vi "Day.vi"() -> ()   [LabVIEW 2021]
uses:
  <vilib>/addons/_JKI Toolkits/Caraya/classes/Assert/Assert Equal Value_Variant.vi
  <vilib>/addons/_JKI Toolkits/Caraya/classes/Assert/Assert.lvclass
  <vilib>/addons/_JKI Toolkits/Caraya/classes/Test/Test.lvclass
panel:
  in  "Input?":enum16{"Examples", "File", "Web"}(ring)=enum."Web"
  in  "Part?":enum16{"Part 1", "Part 2"}(ring)
  out "Solution Part 2":i64
  out "Solution Part 1":i64
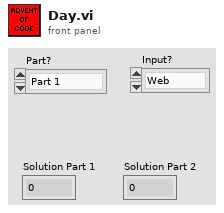
[diagram p1: front panel]
types:
  T1 = cluster{"Result Part1":dbl, "Result Part2":dbl, "Input":string}
  T2 = cluster{"Result Part1":dbl, "Result Part2":dbl, "Input":string}[]
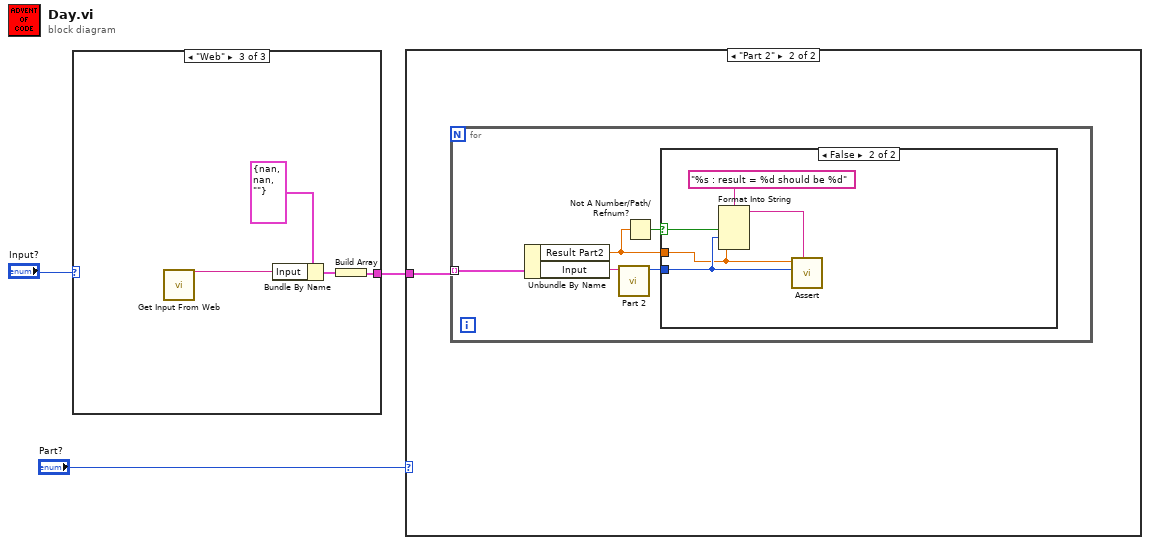
[diagram p0: block diagram]
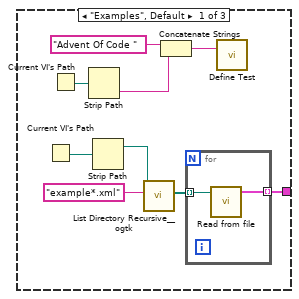
[diagram p2: hidden frame]
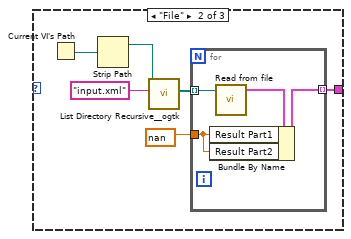
[diagram p3: hidden frame]
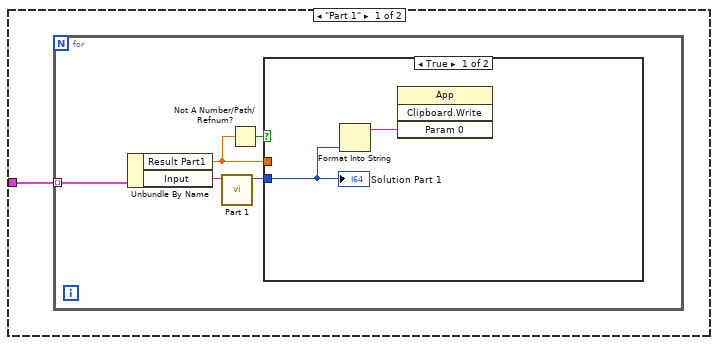
[diagram p4: hidden frame]
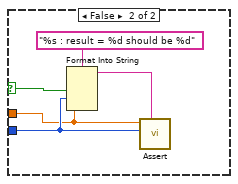
[diagram p5: hidden frame]
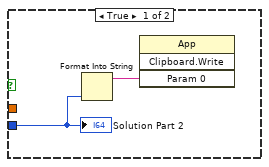
[diagram p6: hidden frame]
diagram:
  n1 = case shown="\"Web\"" "Input?" {
    tunnel: [w8 w16 w26] -> w1
    frame "Examples", Default {
      n2 = Current VI's Path() -> (path=w12:path)
      n3 = Current VI's Path() -> (path=w6:path)
      n4 = Strip Path(path=w6) -> (name=w4:string)  [unwired: 1 out]
      n5 = Strip Path(path=w12) -> (stripped path=w10:path)  [unwired: 1 out]
      n6 = call <userlib>:"List Directory Recursive__ogtk.vi"("pattern"="example*.xml", "Path"=w10) -> ("file paths"=w9:path[])  [unwired: 6 in, 3 out]
      n7 = Concatenate Strings("Advent Of Code " ("Label (VI Title)"), w4) -> (w5:string)
      n8 = for {
        tunnel: w9 -> [w14] mode=indexing
        tunnel: [w13] -> w8 mode=indexing
        n9 = call "Read from file.vi"("File Path"=w14) -> ("Data"=w13:T1)  [unwired: 10 in]
      }
      n10 = call <vilib>:"Define Test.vi"("Label (VI Title)"=w5) -> ()  [unwired: 10 in, 1 out]
    }
    frame "File" {
      n11 = Current VI's Path() -> (path=w20:path)
      n12 = Strip Path(path=w20) -> (stripped path=w18:path)  [unwired: 1 out]
      n13 = call <userlib>:"List Directory Recursive__ogtk.vi"("pattern"="input.xml", "Path"=w18) -> ("file paths"=w17:path[])  [unwired: 6 in, 3 out]
      n14 = for {
        tunnel: w17 -> [w24] mode=indexing
        tunnel: [w22] -> w16 mode=indexing
        tunnel: nan -> [w21]
        n15 = call "Read from file.vi"("File Path"=w24) -> ("Data"=w23:T1)  [unwired: 10 in]
        n16 = Bundle By Name(cluster=w23, "Result Part1"=w21, "Result Part2"=w21) -> (w22:T1)
      }
    }
    frame "Web" {
      n17 = call "Get Input From Web.vi"() -> ("standard output"=w25:string)  [unwired: 11 in]
      n18 = Bundle By Name(cluster=T1 {"Result Part1"=nan, "Result Part2"=nan, "Input"=""} ("Data"), "Input"=w25) -> (w27:T1)
      n19 = Build Array(w27) -> (w26:T2)
    }
  }
  n20 = case shown="\"Part 2\"" "Part?" {
    tunnel: w1 -> [w29 w42]
    frame "Part 1" {
      n21 = for {
        tunnel: w29 -> [w32] mode=indexing
        n22 = Unbundle By Name(w32) -> ("Result Part1"=w30:dbl, "Input"=w34:string)
        n23 = call "Part 1.vi"("Input"=w34) -> ("Output"=w33:i64)  [unwired: 10 in]
        n24 = Not A Number/Path/Refnum?(number/path/refnum=w30) -> (NaN/Path/Refnum?=w31:bool)
        n25 = case shown="True" w31 {
          selector: w31 -> [_ w41]
          tunnel: w30 -> [_ w37]
          tunnel: w33 -> [w35 w38]
          frame True {
            n26 = Format Into String(w35) -> (resulting string=w36:string)  [unwired: 3 in, 1 out]
            n27 = invoke class="App" method="Clipboard.Write"("Param 0"=w36) -> ()  [unwired: 3 in, 4 out]
            "Solution Part 1" <- w35
          }
          frame False {
            n28 = Format Into String(format string="%s : result = %d should be %d", w41, w38, w37) -> (resulting string=w40:string)  [unwired: 2 in, 1 out]
            n29 = call-poly <vilib>:"Assert.vi"("Label"=w40, "Y"=w38, "X"=w37) -> ()  [unwired: 8 in, 1 out]
          }
        }
      }
    }
    frame "Part 2" {
      n30 = for {
        tunnel: w42 -> [w45] mode=indexing
        n31 = Unbundle By Name(w45) -> ("Result Part2"=w43:dbl, "Input"=w47:string)
        n32 = call "Part 2.vi"("Input"=w47) -> ("Output"=w46:i64)  [unwired: 10 in]
        n33 = Not A Number/Path/Refnum?(number/path/refnum=w43) -> (NaN/Path/Refnum?=w44:bool)
        n34 = case shown="False" w44 {
          selector: w44 -> [_ w54]
          tunnel: w43 -> [_ w50]
          tunnel: w46 -> [w49 w51]
          frame True {
            n35 = Format Into String(w49) -> (resulting string=w48:string)  [unwired: 3 in, 1 out]
            n36 = invoke class="App" method="Clipboard.Write"("Param 0"=w48) -> ()  [unwired: 3 in, 4 out]
            "Solution Part 2" <- w49
          }
          frame False {
            n37 = Format Into String(format string="%s : result = %d should be %d", w54, w51, w50) -> (resulting string=w53:string)  [unwired: 2 in, 1 out]
            n38 = call-poly <vilib>:"Assert.vi"("Label"=w53, "Y"=w51, "X"=w50) -> ()  [unwired: 8 in, 1 out]
          }
        }
      }
    }
  }
